vi "Grid_Main_v2.vi"(11 "Settings":T3={"Drift Correction Settings"={"Drift Correction every"=80, "Drift correction Pixels"=256, "Channel index (0-23)"=0, "MaxImagesBack"=2, "Threshold"=2, "Increment"=8, "max applied Drift Correction"=20, "Correct Drift"=TRUE, "Correlate"=0, "Correct z drift"=FALSE, "zdrift \nDuration (s)"=0.0}, "Spectroscopy Setting"={"Imaging Current"=1e-11, "ref Current"=7e-11, "tip Speed (m/s)"=2e-09, "Imaging Bias"=0.02, "ref Bias"=-0.1, "preSTS delay [ms]"=500, "STS z offset"=2e-10, "during Spec Bias (V)"=-0.1, "trigger1 < Hz"=0.0, "trigger 2 >Hz"=0.0, "autoStop"=FALSE, "Spectroscopy"=0, "PLL ON/OFF"=TRUE, "readjust setpoint every "=1, "z Reference (constHeight)"=FALSE, "Lock In"=TRUE}, "Misc"={"File name"="symmetric_node_zOff=200p", "Email when finished"="cornelius.krull@monash.edu,Dhaneesh.Gopalakrishnan@monash.edu,marina.castelli@monash.edu"}, "Grid Settings"={"type"=1, "type order"=1, "X pixel"=0, "Y pixel"=0, "Grid_Parms"={"center X (m)"=0.0, "center Y (m)"=0.0, "width (m)"=0.0, "height (m)"=0.0, "angle (deg)"=0.0}}} {"Grid Settings"."type order" items=["Grid", "Random", "Adam7"]; "Grid Settings"."type" items=["Line", "Grid", "Cloud"]; "Spectroscopy Setting"."Spectroscopy" items=["Bias", "zSpec"]; "Spectroscopy Setting"."trigger 2 >Hz" format="%#_6p"; "Spectroscopy Setting"."trigger1 < Hz" format="%#_6p"; "Spectroscopy Setting"."during Spec Bias (V)" format="%#_5p"; "Spectroscopy Setting"."STS z offset" format="%#_6p"; "Spectroscopy Setting"."ref Bias" format="%#_6p"; "Spectroscopy Setting"."Imaging Bias" format="%#_6p"; "Spectroscopy Setting"."tip Speed (m/s)" format="%.2p"; "Spectroscopy Setting"."ref Current" format="%#_6p"; "Spectroscopy Setting"."Imaging Current" format="%#_6p"; "Drift Correction Settings"."Correlate" items=["first Frame", "successive Frames"]; "Drift Correction Settings"."max applied Drift Correction" min=1 max=100 step=1 format="%.0p"; "Drift Correction Settings"."Threshold" min=1 step=1; "Drift Correction Settings"."Channel index (0-23)" items=["Current"=0, "Z (m)"=14]}) -> (3 "Settings out":T2)   [LabVIEW 2014]
uses:
  <userlib>/Nanonis Prog Interface V5/Nanonis Prog Interface.lvlib
panel:
  in  "resume":T1
  in  "stop":bool
  out "total points":i32
  out "Points taken":i32
  out "ETA":timestamp=timestamp(3575267058.899443 s since 1904-01-01)
  out "remaining time":dbl format="%<%H:%M:%S>t"
  out "Progress":u8(slide)=100 scale=0.0..100.0 scale format="%#.1g"
  out "Last z adjustment":dbl
  out "Last Drift detected (images back)":i32
  out "Y Offset out":sgl format="%#_6p"
  out "X Offset out":sgl format="%#_6p"
  out "Drift Correction Image":picture
  # "RUN smart tilt before starting the GRID\nImg Angle = 0  CHECK CUTOFF\nmove tip to reference point for tip height"
  # "%"
  # "finish the last action and then"
  # "GRID points"
  # "Increase this if no Drift was detected for \na certain number of images"
  # "% of image size"
  # "Only first frame works"
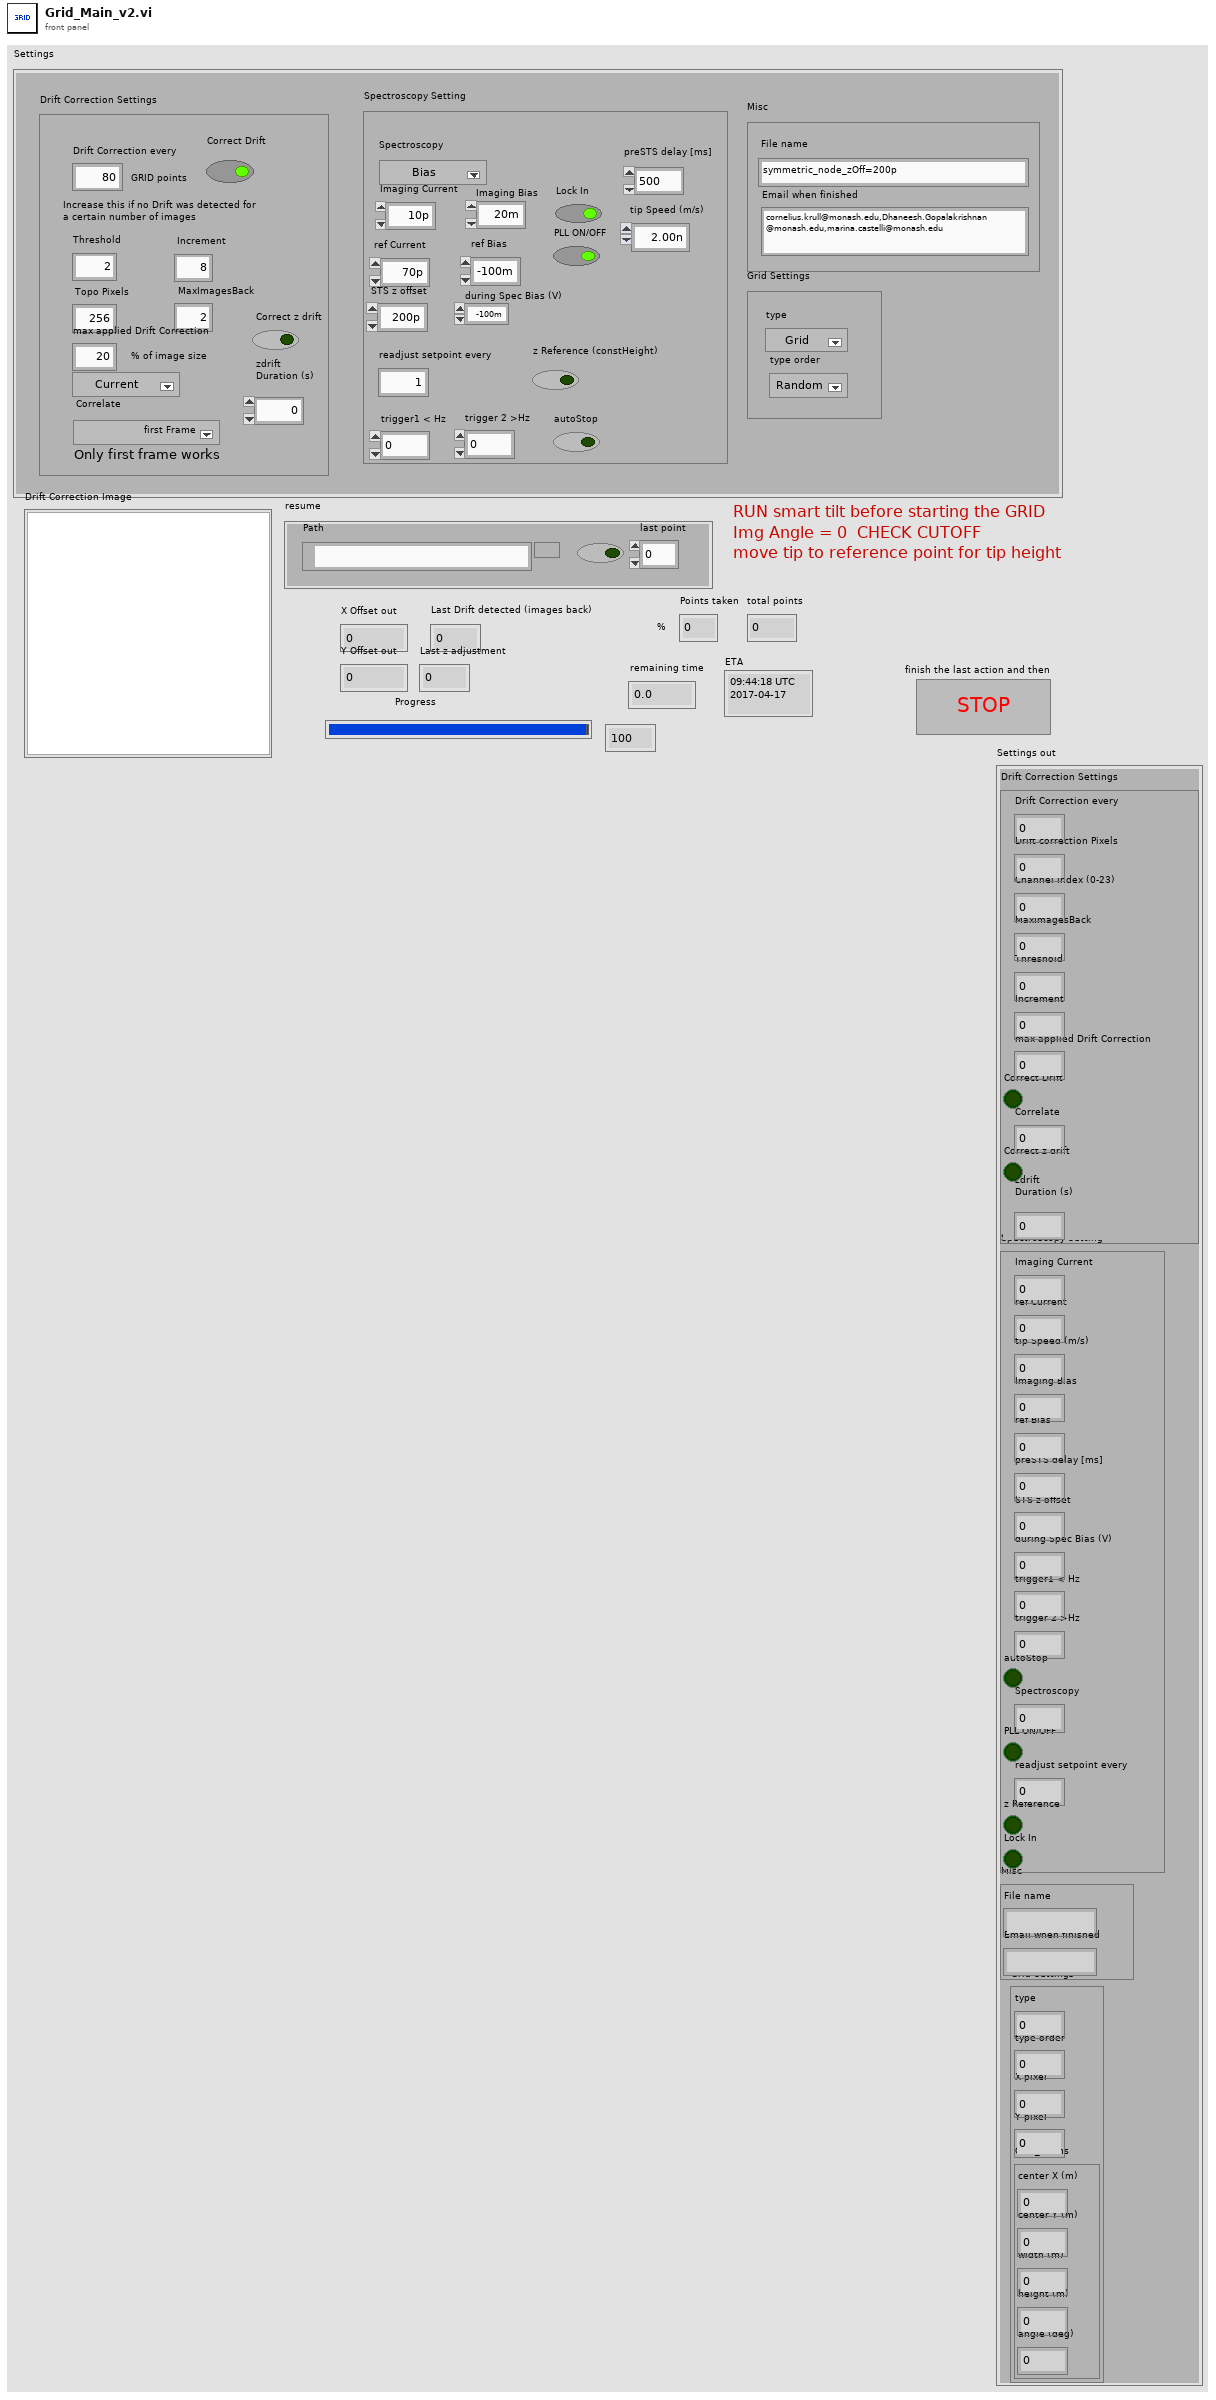
[diagram p1: front panel]
types:
  T1 = cluster{"resume Grid":bool, "Path":path, "last point":i32}
  T2 = cluster{"Drift Correction Settings":cluster{"Drift Correction every":i32, "Drift correction Pixels":i32, "Channel index (0-23)":u8, "MaxImagesBack":i32, "Threshold":i32, "Increment":i32, "max applied Drift Correction":i32, "Correct Drift":bool, "Correlate":u16, "Correct z drift":bool, "zdrift \nDuration (s)":dbl}, "Spectroscopy Setting":cluster{"Imaging Current":dbl, "ref Current":dbl, "tip Speed (m/s)":sgl, "Imaging Bias":dbl, "ref Bias":dbl, "preSTS delay [ms]":u32, "STS z offset":dbl, "during Spec Bias (V)":sgl, "trigger1 < Hz":sgl, "trigger 2 >Hz":sgl, "autoStop":bool, "Spectroscopy":u16, "PLL ON/OFF":bool, "readjust setpoint every ":i32, "z Reference":bool, "Lock In":bool}, "Misc":cluster{"File name":string, "Email when finished":string}, "Grid Settings":cluster{"type":u16, "type order":u16, "X pixel":i32, "Y pixel":i32, "Grid_Parms":cluster{"center X (m)":sgl, "center Y (m)":sgl, "width (m)":sgl, "height (m)":sgl, "angle (deg)":sgl}}}
  T3 = cluster{"Drift Correction Settings":cluster{"Drift Correction every":i32, "Drift correction Pixels":i32, "Channel index (0-23)":u8, "MaxImagesBack":i32, "Threshold":i32, "Increment":i32, "max applied Drift Correction":i32, "Correct Drift":bool, "Correlate":u16, "Correct z drift":bool, "zdrift \nDuration (s)":dbl}, "Spectroscopy Setting":cluster{"Imaging Current":dbl, "ref Current":dbl, "tip Speed (m/s)":sgl, "Imaging Bias":dbl, "ref Bias":dbl, "preSTS delay [ms]":u32, "STS z offset":dbl, "during Spec Bias (V)":sgl, "trigger1 < Hz":sgl, "trigger 2 >Hz":sgl, "autoStop":bool, "Spectroscopy":u16, "PLL ON/OFF":bool, "readjust setpoint every ":i32, "z Reference (constHeight)":bool, "Lock In":bool}, "Misc":cluster{"File name":string, "Email when finished":string}, "Grid Settings":cluster{"type":u16, "type order":u16, "X pixel":i32, "Y pixel":i32, "Grid_Parms":cluster{"center X (m)":sgl, "center Y (m)":sgl, "width (m)":sgl, "height (m)":sgl, "angle (deg)":sgl}}}
  T4 = cluster{"Drift File out":refnum<file>, "zFile":refnum<file>, "BinFile ref":refnum<file>, "xyFile":refnum<file>}
  T5 = cluster{"Drift Correction every":i32, "Drift correction Pixels":i32, "Channel index (0-23)":u8, "MaxImagesBack":i32, "Threshold":i32, "Increment":i32, "max applied Drift Correction":i32, "Correct Drift":bool, "Correlate":u16, "Correct z drift":bool, "zdrift \nDuration (s)":dbl}
  T6 = cluster{"Imaging Current":dbl, "ref Current":dbl, "tip Speed (m/s)":sgl, "Imaging Bias":dbl, "ref Bias":dbl, "preSTS delay [ms]":u32, "STS z offset":dbl, "during Spec Bias (V)":sgl, "trigger1 < Hz":sgl, "trigger 2 >Hz":sgl, "autoStop":bool, "Spectroscopy":u16, "PLL ON/OFF":bool, "readjust setpoint every ":i32, "z Reference":bool, "Lock In":bool}
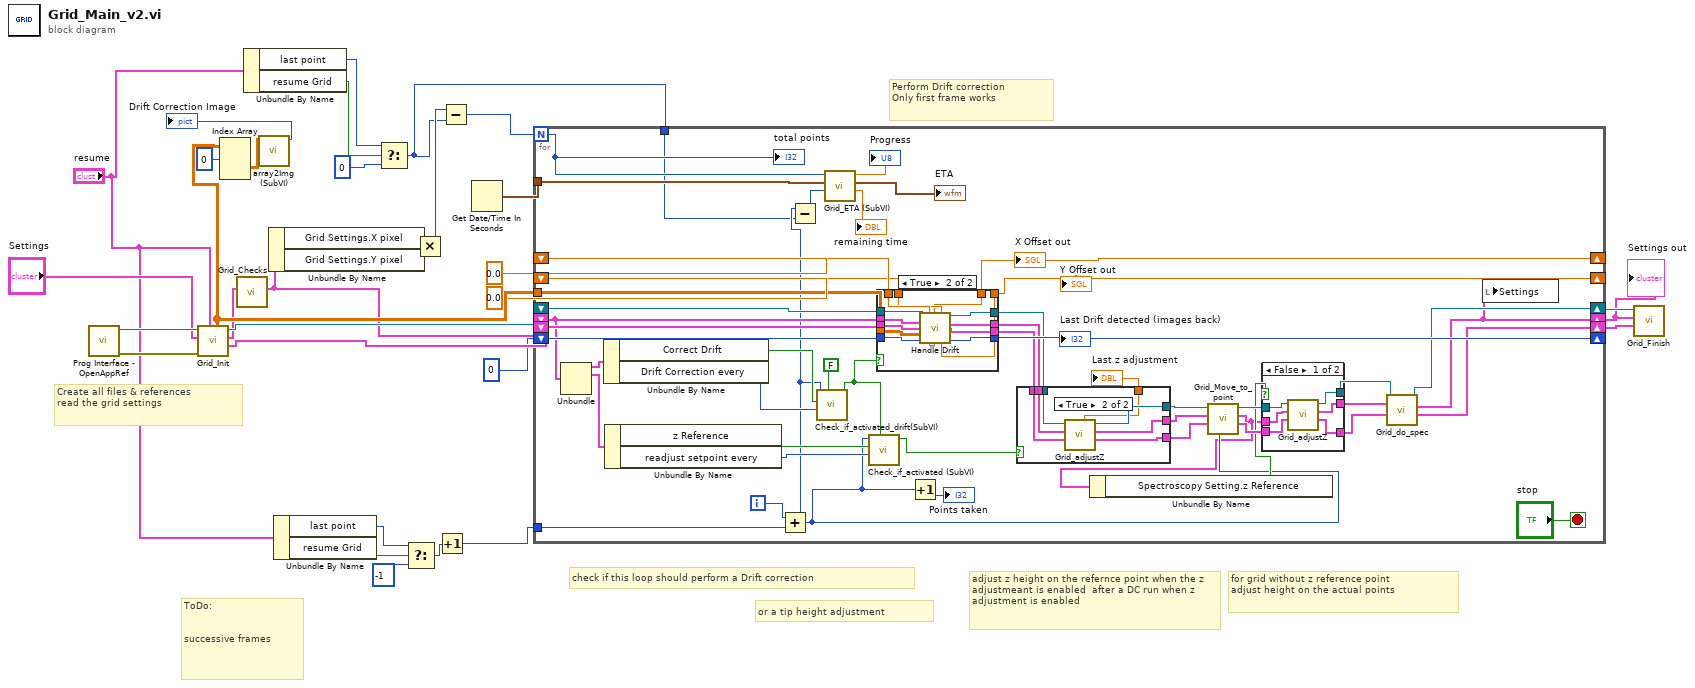
[diagram p0: block diagram]
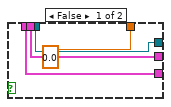
[diagram p3: hidden frame]
diagram:
  # "ToDo:\n\n\nsuccessive frames"
  # "Perform Drift correction\nOnly first frame works"
  # "check if this loop should perform a Drift correction"
  # "for grid without z reference point \nadjust height on the actual points"
  # "or a tip height adjustment"
  # "Create all files & references\nread the grid settings"
  # "adjust z height on the refernce point when the z adjustmeant is enabled  after a DC run when z adjustment is enabled"
  n1 = call <userlib>:"Prog Interface - OpenAppRef.vi"() -> ("Error out"=w31:errorcluster, "Application reference"=w32:refnum<vi>)  [unwired: 6 in]
  n2 = call "Grid_Init.vi"("resume"="resume", "Error in"=w31, "Settings"="Settings", "Application reference"=w32) -> ("FileRefs"=w29:T4, "Settings out"=w15:T2, "Application ref out"=w28:refnum<vi>, "DC images"=w26:dbl[][][])  [unwired: 3 in, 1 out]
  n3 = Index Array(array=w26, index (dim 0)=0 ("index (page)")) -> (element=w27:dbl[][])  [unwired: 2 in]
  n4 = call "Grid_Checks.vi"("Settings"=w15) -> ("Settings out"=w14:T2)  [unwired: 10 in]
  n5 = Unbundle By Name("resume") -> ("last point"=w4:i32, "resume Grid"=w6:bool)
  n6 = call "array2Img (SubVI).vi"("Rxy"=w27) -> ("new picture"=→"Drift Correction Image":picture)  [unwired: 10 in]
  n7 = Unbundle By Name(w14) -> ("Grid Settings.X pixel"=w21:i32, "Grid Settings.Y pixel"=w20:i32)
  n8 = Unbundle By Name("resume") -> ("last point"=w10:i32, "resume Grid"=w12:bool)
  n9 = Select(t=w4, s=w6, f=0) -> (s? t:f=w1:i32)
  n10 = Select(t=w10, s=w12, f=-1) -> (s? t:f=w9:i32)
  n11 = Multiply(x=w21, y=w20) -> (x*y=w2:i32)
  n12 = Increment(x=w9) -> (x+1=w7:i32)
  n13 = Subtract(x=w2, y=w1) -> (x-y=w8:i32)
  n14 = Get Date/Time In Seconds() -> (seconds since 1Jan1904=w19:timestamp)
  n15 = for {
    N: w8 -> [w38]
    tunnel: w26 -> [w78]
    shift-right: [w77] -> _
    shift-left: 0 ("Last Drift out") -> [w76]
    shift-right: [w72] -> _
    shift-left: sgl 0.0 ("X Offset out") -> [w75]
    shift-right: [w73] -> _
    shift-left: sgl 0.0 ("Y Offset out") -> [w74]
    tunnel: w19 -> [w63]
    shift-right: [w60] -> w18
    shift-left: w28 -> [w79]
    shift-right: [w34] -> w17
    shift-left: w14 -> [w45]
    shift-right: [w59] -> w16
    shift-left: w29 -> [w80]
    tunnel: w7 -> [w46]
    tunnel: w1 -> [w35]
    i -> [w57]
    stop <- "stop" stop-if-true
    n16 = Unbundle(w45) -> ("Drift Correction Settings"=w44:T5, "Spectroscopy Setting"=w42:T6)  [unwired: 2 out]
    n17 = Unbundle By Name(w44) -> ("Correct Drift"=w43:bool, "Drift Correction every"=w39:i32)
    n18 = Unbundle By Name(w42) -> ("z Reference"=w41:bool, "readjust setpoint every"=w40:i32)
    n19 = Add(x=w57, y=w46) -> (x+y=w36:i32)
    n20 = Subtract(x=w36, y=w35) -> (x-y=w37:i32)
    n21 = call "Check_if_activated_drift(SubVI).vi"("Override"=FALSE, "activate  every  iterations"=w39, "activated?"=w43, "Iteration"=w36) -> ("perform action"=w68:bool)  [unwired: 7 in]
    n22 = call "Grid_ETA (SubVI).vi"("points taken"=w37, "seconds since 1Jan1904"=w63, "points todo"=w38) -> ("Numeric 4"=→"remaining time":dbl, "Time Stamp"=→"ETA":timestamp, "Numeric 3"=→"Progress":dbl)  [unwired: 6 in]
    n23 = call "Check_if_activated (SubVI).vi"("Override"=w68, "activate  every  iterations"=w40, "activated?"=w41, "Iteration"=w36) -> ("perform action"=w69:bool)  [unwired: 7 in]
    n24 = case shown="True" w68 {
      tunnel: w45 -> [w103 w119]
      tunnel: w80 -> [w102 w118]
      tunnel: w79 -> [w101 w117]
      tunnel: w78 -> [_ w116]
      tunnel: [w104 w115] -> w77
      tunnel: w76 -> [w104 w114]
      tunnel: w75 -> [w106 w113]
      tunnel: w74 -> [w105 w112]
      tunnel: [w105 w111] -> w73
      tunnel: [w106 w110] -> w72
      tunnel: [w101 w109] -> w71
      tunnel: [w103 w108] -> w48
      tunnel: [w102 w107] -> w70
      frame False {
      }
      frame True {
        n25 = call "Handle Drift.vi"("Application ref in"=w117, "X Offset in"=w113, "Y Offset In"=w112, "Settings"=w119, "FileRefs"=w118, "Drift Correction image"=w116, "Last Drift"=w114) -> ("Application out"=w109:refnum<vi>, "Settings out"=w108:T2, "FileRefs out File Refs  Out"=w107:T4, "X Offset out"=w110:sgl, "Y Offset out"=w111:sgl, "Last Drift out"=w115:i32)  [unwired: 3 in]
      }
    }
    "X Offset out" <- w72
    "Y Offset out" <- w73
    "Last Drift detected (images back)" <- w77
    n26 = Increment(x=w36) -> (x+1=→"Points taken":i32)
    n27 = case shown="True" w69 {
      tunnel: w71 -> [w92 w100]
      tunnel: w70 -> [w91 w99]
      tunnel: w48 -> [w90 w98]
      tunnel: [w91 w97] -> w62
      tunnel: [w90 w96] -> w50
      tunnel: [w92 w95] -> w61
      tunnel: [0.0 ("Last z adjustment") w94] -> w58
      frame False {
      }
      frame True {
        n28 = call "Grid_adjustZ.vi"("FileRefs"=w99, "Settings"=w98, "Application in"=w100) -> ("FileRefs out"=w97:T4, "Settings out"=w96:T2, "Application ref out"=w95:refnum<vi>, "Last z adjustment"=w94:dbl)  [unwired: 4 in, 1 out]
      }
    }
    "Last z adjustment" <- w58
    n29 = call "Grid_Move_to_point.vi"("point"=w36, "FileRefs in"=w62, "Settings"=w50, "Application ref in"=w61) -> ("FileRefs out"=w52:T4, "Settings out"=w33:T2, "Application ref out"=w53:refnum<vi>)  [unwired: 5 in]
    n30 = Unbundle By Name(w33) -> ("Spectroscopy Setting.z Reference"=w51:bool)
    n31 = case shown="False" w51 {
      tunnel: [w86 w89] -> w56
      tunnel: [w85 w87] -> w54
      tunnel: [w84 w88] -> w55
      tunnel: w53 -> [w83 w89]
      tunnel: w33 -> [w82 w88]
      tunnel: w52 -> [w81 w87]
      frame False {
        n32 = call "Grid_adjustZ.vi"("FileRefs"=w81, "Settings"=w82, "Application in"=w83) -> ("FileRefs out"=w85:T4, "Settings out"=w84:T2, "Application ref out"=w86:refnum<vi>)  [unwired: 4 in, 2 out]
      }
      frame True {
      }
    }
    n33 = call "Grid_do_spec.vi"("FileRefs in"=w54, "Settings in"=w55, "Application ref in"=w56) -> ("FileRefs out"=w59:T4, "Settings out"=w34:T2, "Application ref out"=w60:refnum<vi>)  [unwired: 5 in, 1 out]
    n34 = local write "Settings"(w34) -> ()
    "total points" <- w38
  }
  "Settings out" <- w17
  n35 = call "Grid_Finish.vi"("FileRefs"=w16, "Settings"=w17, "Application reference"=w18) -> ()  [unwired: 9 in]
